vi "StopRecordSpecialMarlin.vi"(4 "error in (no error)":errorcluster, 6 "ClusterRefCtrlIN":T1, 7 "task/channels in":refnum<k21>) -> (0 "error out":errorcluster, 2 "RecStopped":bool, 3 "task out":refnum<k21>)   [LabVIEW 2015]
uses:
  DefDeType/ClusterRefCtrl.ctl
  <vilib>/DAQmx/write.llb/DAQmx Write (Digital Bool 1Line 1Point).vi
  <vilib>/DAQmx/miscellaneous.llb/DAQmx Fill In Error Info.vi
  Globals/NortekInstruction.vi
  Globals/QualisysInstruction.vi
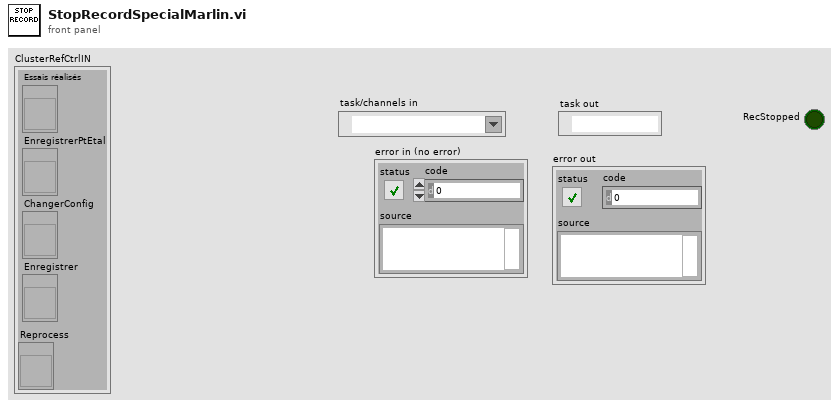
[diagram p1: front panel]
types:
  T1 = typedef "ClusterRefCtrl.ctl" = cluster{"Essais réalisés":refnum<vi>, "EnregistrerPtEtal":refnum<vi>, "ChangerConfig":refnum<vi>, "Enregistrer":refnum<vi>, "Reprocess":refnum<vi>}
  T2 = enum8{"Enabled", "Disabled", "Disabled and Grayed Out"}
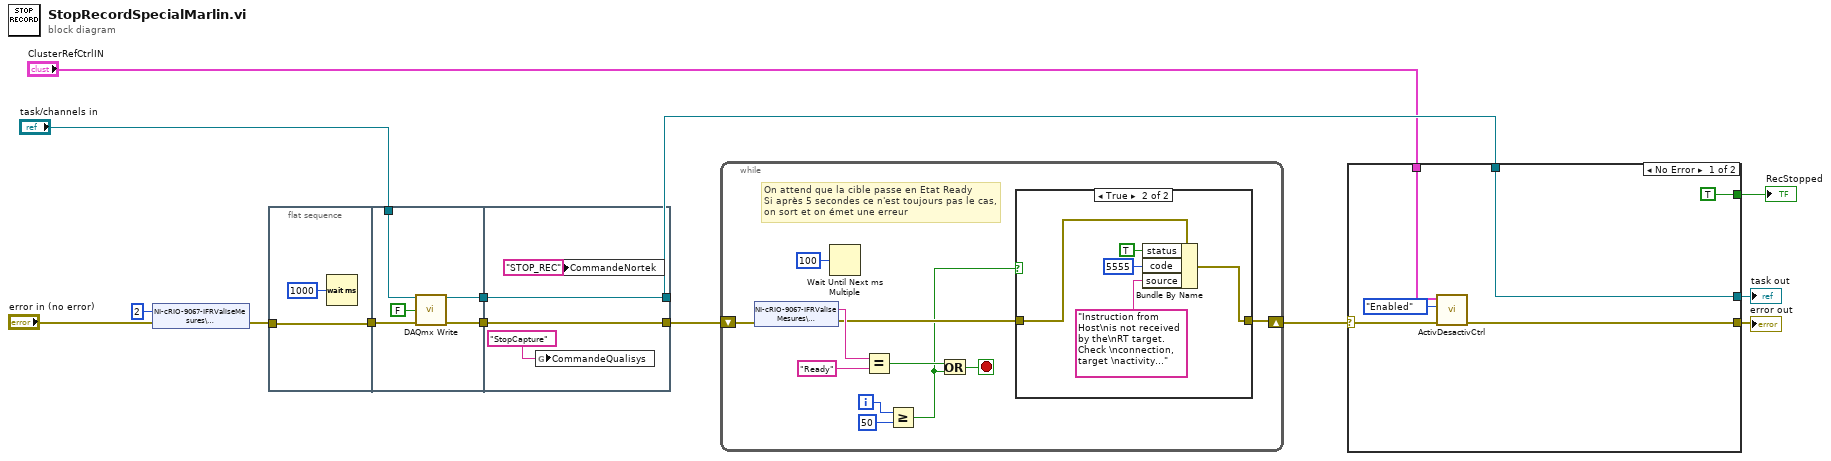
[diagram p0: block diagram]
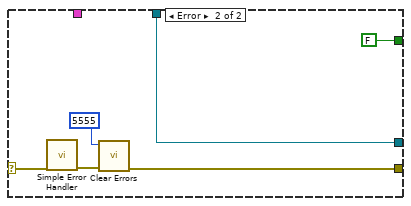
[diagram p2: hidden frame]
diagram:
  n1 = shared-variable "NI-cRIO-9067-IFRValiseMesures\\Bibliothèque2Variables.lvlib\\Instruction"(u8 2 ("Instruction"), error in="error in (no error)") -> (error out=w7:errorcluster)
  n2 = flat-sequence {
    tunnel: w7 -> [w15]
    tunnel: [w15] -> w8
    tunnel: w8 -> [w20]
    tunnel: "task/channels in" -> [w18]
    tunnel: [w19] -> w3
    tunnel: [w17] -> w2
    tunnel: [w24] -> w4
    tunnel: [w25] -> w6
    tunnel: w3 -> [w25]
    tunnel: w2 -> [w24]
    frame #0 {
      n3 = Wait (ms)(milliseconds to wait=u32 1000) -> ()  [unwired: 1 out]
    }
    frame #1 {
      n4 = call-poly <vilib>:"DAQmx Write.vi"("task/channels in"=w18, "data"=FALSE, "error in"=w20) -> ("task out"=w17:refnum<k21>, "error out"=w19:errorcluster)  [unwired: 10 in, 1 out]
    }
    frame #2 {
      n5 = global write "QualisysInstruction.vi" "CommandeQualisys"("StopCapture" ("Command")) -> ()
      n6 = global write "NortekInstruction.vi" "CommandeNortek"("STOP_REC" ("Command")) -> ()
    }
  }
  n7 = while {
    shift-right: [w26] -> w12
    shift-left: w6 -> [w36]
    i -> [w32]
    stop <- w29 stop-if-true
    # "On attend que la cible passe en Etat Ready\nSi après 5 secondes ce n'est toujours pas le cas, \non sort et on émet une erreur"
    n8 = shared-variable "NI-cRIO-9067-IFRValiseMesures\\Bibliothèque2Variables.lvlib\\RTState"(error in=w36) -> (w35:string, error out=w28:errorcluster)
    n9 = Wait Until Next ms Multiple(millisecond multiple=u32 100) -> ()  [unwired: 1 out]
    n10 = Equal?(x=w35, y="Ready") -> (x = y?=w30:bool)
    n11 = Greater Or Equal?(x=w32, y=50) -> (x >= y?=w27:bool)
    n12 = Or(x=w30, y=w27) -> (x .or. y?=w29:bool)
    n13 = case shown="True" w27 {
      tunnel: w28 -> [w37 w42]
      tunnel: [w37 w38] -> w26
      frame False {
      }
      frame True {
        n14 = Bundle By Name(cluster=w42, "status"=TRUE, "code"=5555, "source"="Instruction from Host\nis not received by the\nRT target. Check \nconnection, target \nactivity...") -> (w38:errorcluster)
      }
    }
  }
  n15 = case shown="No Error" w12 {
    selector: w12 -> [w46 w53]
    tunnel: w4 -> [w47 w54]
    tunnel: [w45 w50] -> w10
    tunnel: [w47 w54] -> w11
    tunnel: [TRUE ("RecStarted") FALSE ("RecStarted")] -> w9
    tunnel: "ClusterRefCtrlIN" -> [w43 _]
    frame No Error {
      n16 = call "ActivDesactivCtrl.vi"("error in (no error)"=w46, "Disabled"=T2."Enabled", "Cluster"=w43) -> ("error out"=w45:errorcluster)  [unwired: 4 in]
    }
    frame Error {
      n17 = call <vilib>:"Simple Error Handler.vi"("error in (no error)"=w53) -> ("error out"=w52:errorcluster)  [unwired: 4 in, 4 out]
      n18 = call <vilib>:"Clear Errors.vi"("error in (no error)"=w52, "specific error code to clear (0: all)"=5555) -> ("error out"=w50:errorcluster)  [unwired: 4 in, 1 out]
    }
  }
  "task out" <- w11
  "error out" <- w10
  "RecStopped" <- w9
